vi "Read Control.vi"(5 "section":string, 7 "Prefix":string, 8 "Error In":errorcluster, 10 "File refnum":T1, 11 "Ctl Refnum":refnum<vi>) -> (0 "Error Out":errorcluster, 3 "Ctl Refnum out":refnum<vi>)   [LabVIEW 2015]
uses:
  <vilib>/Utility/Data Type/NI_Data Type.lvlib
  <vilib>/Utility/config.llb/NI_LVConfig.lvlib
  <vilib>/Utility/config.llb/Read Key (U32).vi
  <vilib>/Utility/config.llb/Read Key (Double).vi
  <vilib>/Utility/config.llb/Read Key (I32).vi
  <vilib>/Utility/config.llb/Read Key (Boolean).vi
  <vilib>/Utility/config.llb/Read Key (String).vi
  <vilib>/Utility/config.llb/Read Key (Path).vi
  <vilib>/Utility/config.llb/Config Data RefNum.ctl
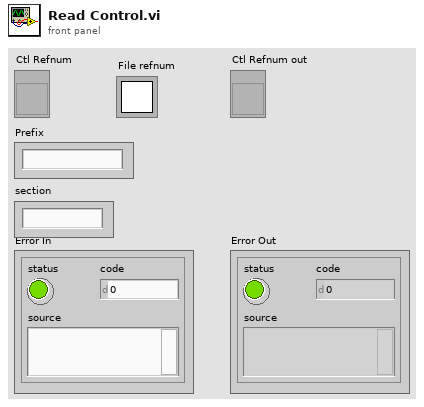
[diagram p1: front panel]
types:
  T1 = typedef "NI_LVConfig.lvlib/Config Data RefNum.ctl" = refnum<k1>
  T2 = typedef "NI_Data Type.lvlib/Data Type.ctl" = enum8{"Invalid Type", "Void", "I8", "I16", "I32", "I64", "U8", "U16", "U32", "U64", "Single Float", "Double Float", "Extended Float", "Single Complex", "Double Complex", "Extended Complex", "Enum U8", "Enum U16", "Enum U32", "Enum U64", "Single Float With Unit", "Double Float With Unit", "Extended Float With Unit", "Single Complex with Unit", "Double Complex with Unit", "Extended Complex with Unit", "Boolean", "String", "Path", "Picture", "Tag", "Array", "Cluster", "Variant", "LV Variant", "Waveform", "Timestamp", "Digital Waveform", "Digital Data", "ExpressData", "Refnum", "External Data", "VI", "Poly VI", "LabVIEW Class Instance", "Fixed Point"}
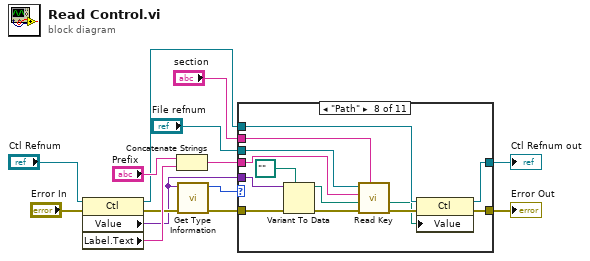
[diagram p0: block diagram]
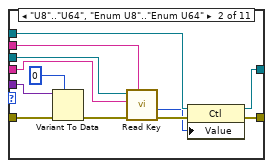
[diagram p3: hidden frame]
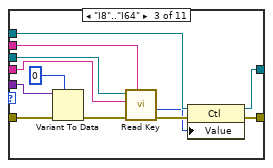
[diagram p4: hidden frame]
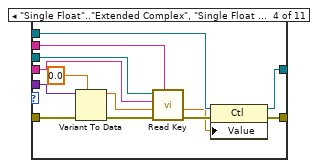
[diagram p5: hidden frame]
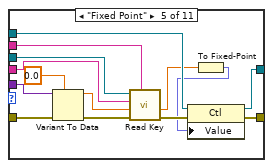
[diagram p6: hidden frame]
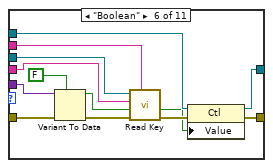
[diagram p7: hidden frame]
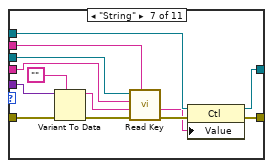
[diagram p8: hidden frame]
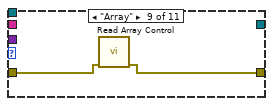
[diagram p9: hidden frame]
diagram:
  n1 = property class="Ctl"(reference="Ctl Refnum", error in="Error In") -> (reference out=w7:refnum<vi>, error out=w6:errorcluster, "Value"=w1:variant, "Label.Text"=w10:string)
  n2 = Concatenate Strings("Prefix", w10) -> (w8:string)
  n3 = call <vilib>:"Get Type Information.vi"("error in (no error)"=w6, "Variant"=w1) -> ("error out"=w5:errorcluster, "Type"=w13:T2)  [unwired: 5 in, 3 out]
  n4 = case shown="\"Path\"" w13 {
    tunnel: "File refnum" -> [_ w28 w40 w53 w67 w80 w93 w106 _ _ _]
    tunnel: "section" -> [_ w27 w39 w52 w66 w79 w92 w105 _ _ _]
    tunnel: w8 -> [_ w26 w38 w51 w65 w78 w91 w104 _ _ _]
    tunnel: w7 -> [w15 w25 w37 w50 w64 w77 w90 w103 _ _ _]
    tunnel: w5 -> [w16 w18 w31 w44 w59 w71 w84 w97 w108 _ _]
    tunnel: [w15 w22 w34 w47 w62 w74 w87 w100 _ _ _] -> w4
    tunnel: [w16 w21 w33 w46 w61 w73 w86 w99 w107 _ _] -> w3
    tunnel: w1 -> [_ w17 w29 w45 w60 w72 w85 w98 _ _ _]
    frame "Invalid Type", Default {
    }
    frame "U8".."U64", "Enum U8".."Enum U64" {
      n5 = Variant To Data(error in=w18, type=u32 0, Variant=w17) -> (error out=w19:errorcluster)  [unwired: 1 out]
      n6 = call-poly <vilib>:"Read Key.vi"("section"=w27, "error in (no error)"=w19, "key"=w26, "refnum"=w28) -> ("error out"=w24:errorcluster, "value"=w23:u32)  [unwired: 4 in, 2 out]
      n7 = property class="Ctl"(reference=w25, error in=w24, "Value"=w23) -> (reference out=w22:refnum<vi>, error out=w21:errorcluster)
    }
    frame "I8".."I64" {
      n8 = Variant To Data(error in=w31, type=0, Variant=w29) -> (error out=w30:errorcluster)  [unwired: 1 out]
      n9 = call-poly <vilib>:"Read Key.vi"("section"=w39, "error in (no error)"=w30, "key"=w38, "refnum"=w40) -> ("error out"=w36:errorcluster, "value"=w35:i32)  [unwired: 4 in, 2 out]
      n10 = property class="Ctl"(reference=w37, error in=w36, "Value"=w35) -> (reference out=w34:refnum<vi>, error out=w33:errorcluster)
    }
    frame "Single Float".."Extended Complex", "Single Float With Unit".."Extended Complex with Unit" {
      n11 = Variant To Data(error in=w44, type=0.0, Variant=w45) -> (data=w42:dbl, error out=w43:errorcluster)
      n12 = call-poly <vilib>:"Read Key.vi"("section"=w52, "error in (no error)"=w43, "default value"=w42, "key"=w51, "refnum"=w53) -> ("error out"=w49:errorcluster, "value"=w48:dbl)  [unwired: 3 in, 2 out]
      n13 = property class="Ctl"(reference=w50, error in=w49, "Value"=w48) -> (reference out=w47:refnum<vi>, error out=w46:errorcluster)
    }
    frame "Fixed Point" {
      n14 = Variant To Data(error in=w59, type=0.0, Variant=w60) -> (data=w57:dbl, error out=w58:errorcluster)
      n15 = call-poly <vilib>:"Read Key.vi"("section"=w66, "error in (no error)"=w58, "default value"=w57, "key"=w65, "refnum"=w67) -> ("error out"=w63:errorcluster, "value"=w55:dbl)  [unwired: 3 in, 2 out]
      n16 = To Fixed-Point(number=w55) -> (fixed-point=w54:fxp<+/-,32,16>)  [unwired: 1 in]
      n17 = property class="Ctl"(reference=w64, error in=w63, "Value"=w54) -> (reference out=w62:refnum<vi>, error out=w61:errorcluster)
    }
    frame "Boolean" {
      n18 = Variant To Data(error in=w71, type=FALSE, Variant=w72) -> (data=w69:bool, error out=w70:errorcluster)
      n19 = call-poly <vilib>:"Read Key.vi"("section"=w79, "error in (no error)"=w70, "default value"=w69, "key"=w78, "refnum"=w80) -> ("error out"=w76:errorcluster, "value"=w75:bool)  [unwired: 3 in, 2 out]
      n20 = property class="Ctl"(reference=w77, error in=w76, "Value"=w75) -> (reference out=w74:refnum<vi>, error out=w73:errorcluster)
    }
    frame "String" {
      n21 = Variant To Data(error in=w84, type="", Variant=w85) -> (data=w82:string, error out=w83:errorcluster)
      n22 = call-poly <vilib>:"Read Key.vi"("section"=w92, "error in (no error)"=w83, "default value"=w82, "key"=w91, "refnum"=w93) -> ("error out"=w89:errorcluster, "value"=w88:string)  [unwired: 3 in, 2 out]
      n23 = property class="Ctl"(reference=w90, error in=w89, "Value"=w88) -> (reference out=w87:refnum<vi>, error out=w86:errorcluster)
    }
    frame "Path" {
      n24 = Variant To Data(error in=w97, type=path "", Variant=w98) -> (data=w95:path, error out=w96:errorcluster)
      n25 = call-poly <vilib>:"Read Key.vi"("section"=w105, "error in (no error)"=w96, "default value"=w95, "key"=w104, "refnum"=w106) -> ("error out"=w102:errorcluster, "value"=w101:path)  [unwired: 3 in, 2 out]
      n26 = property class="Ctl"(reference=w103, error in=w102, "Value"=w101) -> (reference out=w100:refnum<vi>, error out=w99:errorcluster)
    }
    frame "Array" {
      n27 = call "Read Array Control.vi"("Error In"=w108) -> ("Error Out"=w107:errorcluster)  [unwired: 8 in, 2 out]
    }
    frame "Cluster" {
    }
    frame "Fixed Point" {
    }
  }
  "Ctl Refnum out" <- w4
  "Error Out" <- w3
